vi "Meas Result Generate TWM Correction - Parametric Uncertainty Set Captions.vi"(7 "correction type":T1, 8 "error in (no error)":errorcluster, 11 "unc params":T2) -> (0 "error out":errorcluster)   [LabVIEW 2020]
doc: "Sets controls formats and captions for parametric uncertainty generator."
uses:
  Meas Results TWM Correction Uncertainty Parametric Generator Ctrls.ctl
  Meas Results TWM Correction Uncertainty Parametric Generator Type.ctl
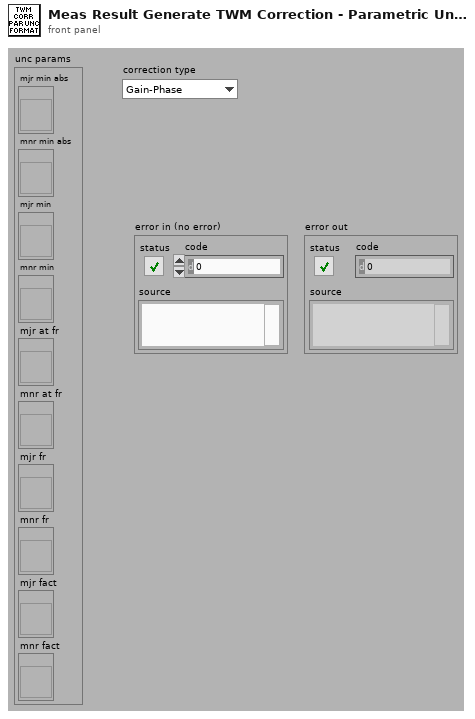
[diagram p1: front panel]
types:
  T1 = typedef "Meas Results TWM Correction Uncertainty Parametric Generator Type.ctl" = enum16{"Gain-Phase", "Cp-Gp", "Rs-Ls"}
  T2 = typedef "Meas Results TWM Correction Uncertainty Parametric Generator Ctrls.ctl" = cluster{"mjr min abs":refnum<vi>, "mnr min abs":refnum<vi>, "mjr min":refnum<vi>, "mnr min":refnum<vi>, "mjr at fr":refnum<vi>, "mnr at fr":refnum<vi>, "mjr fr":refnum<vi>, "mnr fr":refnum<vi>, "mjr fact":refnum<vi>, "mnr fact":refnum<vi>}
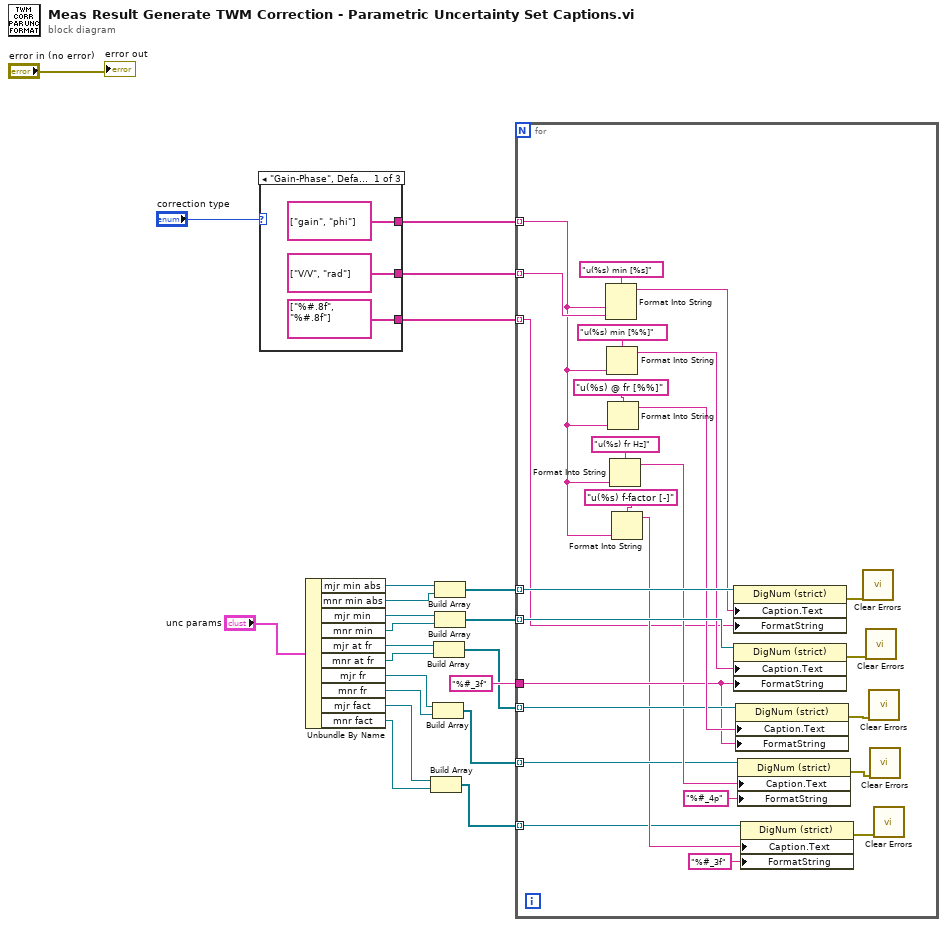
[diagram p0: block diagram]
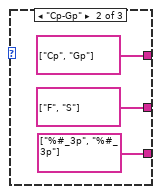
[diagram p2: hidden frame]
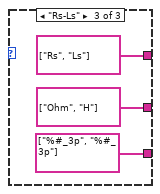
[diagram p3: hidden frame]
diagram:
  n1 = case shown="\"Gain-Phase\", Default" "correction type" {
    tunnel: [string[] ["gain", "phi"] string[] ["Cp", "Gp"] string[] ["Rs", "Ls"]] -> w18
    tunnel: [string[] ["V/V", "rad"] string[] ["F", "S"] string[] ["Ohm", "H"]] -> w17
    tunnel: [string[] ["%#.8f", "%#.8f"] string[] ["%#_3p", "%#_3p"] string[] ["%#_3p", "%#_3p"]] -> w15
    frame "Gain-Phase", Default {
    }
    frame "Cp-Gp" {
    }
    frame "Rs-Ls" {
    }
  }
  n2 = Unbundle By Name("unc params") -> ("mjr min abs"=w20:refnum<vi>, "mnr min abs"=w19:refnum<vi>, "mjr min"=w14:refnum<vi>, "mnr min"=w13:refnum<vi>, "mjr at fr"=w10:refnum<vi>, "mnr at fr"=w9:refnum<vi>, "mjr fr"=w7:refnum<vi>, "mnr fr"=w6:refnum<vi>, "mjr fact"=w4:refnum<vi>, "mnr fact"=w3:refnum<vi>)
  n3 = Build Array(w4, w3) -> (w2:refnum<vi>[])
  n4 = Build Array(w7, w6) -> (w5:refnum<vi>[])
  n5 = Build Array(w10, w9) -> (w8:refnum<vi>[])
  n6 = Build Array(w20, w19) -> (w16:refnum<vi>[])
  n7 = Build Array(w14, w13) -> (w12:refnum<vi>[])
  n8 = for {
    tunnel: w18 -> [w51] mode=indexing
    tunnel: w17 -> [w57] mode=indexing
    tunnel: w16 -> [w50] mode=indexing
    tunnel: w15 -> [w32] mode=indexing
    tunnel: w12 -> [w48] mode=indexing
    tunnel: "%#_3f" ("Format String") -> [w44]
    tunnel: w8 -> [w45] mode=indexing
    tunnel: w5 -> [w42] mode=indexing
    tunnel: w2 -> [w39] mode=indexing
    n9 = Format Into String(format string="u(%s) min [%s]", w51, w57) -> (resulting string=w49:string)  [unwired: 2 in, 1 out]
    n10 = Format Into String(format string="u(%s) min [%%]", w51) -> (resulting string=w47:string)  [unwired: 2 in, 1 out]
    n11 = Format Into String(format string="u(%s) @ fr [%%]", w51) -> (resulting string=w46:string)  [unwired: 2 in, 1 out]
    n12 = Format Into String(format string="u(%s) fr Hz]", w51) -> (resulting string=w43:string)  [unwired: 2 in, 1 out]
    n13 = Format Into String(format string="u(%s) f-factor [-]", w51) -> (resulting string=w40:string)  [unwired: 2 in, 1 out]
    n14 = property class="DigNum (strict)"(reference=w50, "Caption.Text"=w49, "FormatString"=w32) -> (error out=w37:errorcluster)  [unwired: 1 in, 1 out]
    n15 = property class="DigNum (strict)"(reference=w48, "Caption.Text"=w47, "FormatString"=w44) -> (error out=w36:errorcluster)  [unwired: 1 in, 1 out]
    n16 = property class="DigNum (strict)"(reference=w45, "Caption.Text"=w46, "FormatString"=w44) -> (error out=w35:errorcluster)  [unwired: 1 in, 1 out]
    n17 = property class="DigNum (strict)"(reference=w42, "Caption.Text"=w43, "FormatString"="%#_4p" ("Format String")) -> (error out=w34:errorcluster)  [unwired: 1 in, 1 out]
    n18 = property class="DigNum (strict)"(reference=w39, "Caption.Text"=w40, "FormatString"="%#_3f" ("Format String")) -> (error out=w33:errorcluster)  [unwired: 1 in, 1 out]
    n19 = call <vilib>:"Clear Errors.vi"("error in (no error)"=w37) -> ()  [unwired: 5 in, 2 out]
    n20 = call <vilib>:"Clear Errors.vi"("error in (no error)"=w36) -> ()  [unwired: 5 in, 2 out]
    n21 = call <vilib>:"Clear Errors.vi"("error in (no error)"=w35) -> ()  [unwired: 5 in, 2 out]
    n22 = call <vilib>:"Clear Errors.vi"("error in (no error)"=w34) -> ()  [unwired: 5 in, 2 out]
    n23 = call <vilib>:"Clear Errors.vi"("error in (no error)"=w33) -> ()  [unwired: 5 in, 2 out]
  }
  "error out" <- "error in (no error)"
